vi "Set Aircraft Extra Data.vi"(7 "Aircraft ID":u8, 8 "Error In":errorcluster, 11 "Extra Data In":T1) -> (0 "Error Out":errorcluster, 3 "Extra Data Out":T1)   [LabVIEW 2014]
uses:
  Controls/Aircraft Extra Data.ctl
  MAVLink/Controls/MAVLink Optical Flow.ctl
  MAVLink/Controls/MAVLink EKF Status Report.ctl
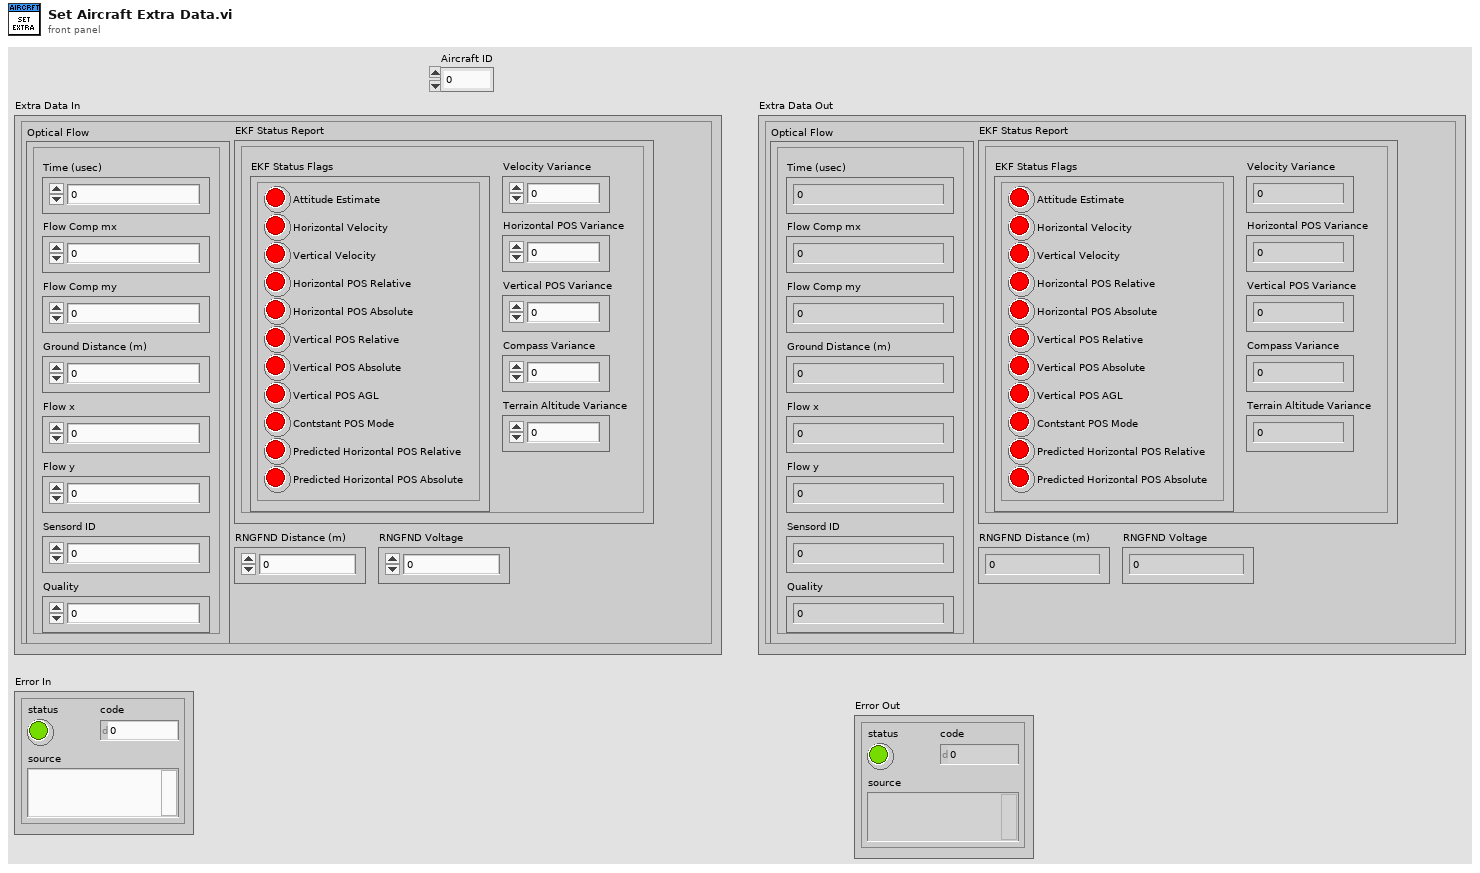
[diagram p1: front panel]
types:
  T1 = typedef "Aircraft Extra Data.ctl" = cluster{"Optical Flow":T2, "RNGFND Distance (m)":sgl, "RNGFND Voltage":sgl, "EKF Status Report":T3}
  T2 = typedef "MAVLink Optical Flow.ctl" = cluster{"Time (usec)":u64, "Flow Comp mx":sgl, "Flow Comp my":sgl, "Ground Distance (m)":sgl, "Flow x":i16, "Flow y":i16, "Sensord ID":u8, "Quality":u8}
  T3 = typedef "MAVLink EKF Status Report.ctl" = cluster{"EKF Status Flags":cluster{"Attitude Estimate":bool, "Horizontal Velocity":bool, "Vertical Velocity":bool, "Horizontal POS Relative":bool, "Horizontal POS Absolute":bool, "Vertical POS Relative":bool, "Vertical POS Absolute":bool, "Vertical POS AGL":bool, "Contstant POS Mode":bool, "Predicted Horizontal POS Relative":bool, "Predicted Horizontal POS Absolute":bool}, "Velocity Variance":sgl, "Horizontal POS Variance":sgl, "Vertical POS Variance":sgl, "Compass Variance":sgl, "Terrain Altitude Variance":sgl}
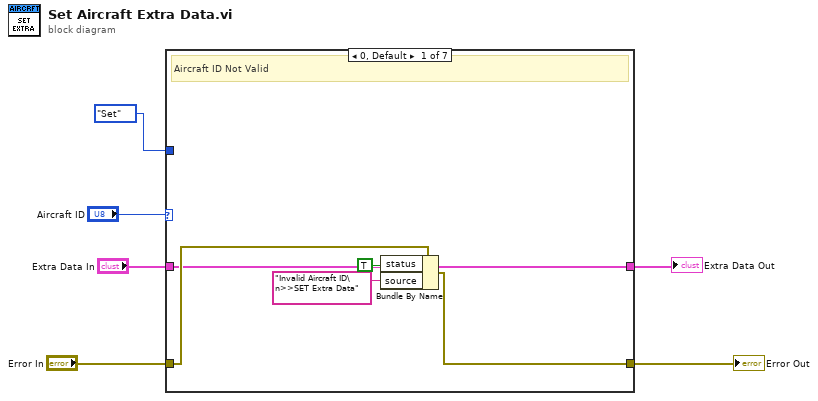
[diagram p0: block diagram]
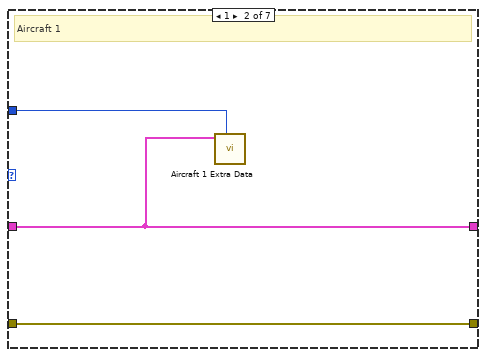
[diagram p2: hidden frame]
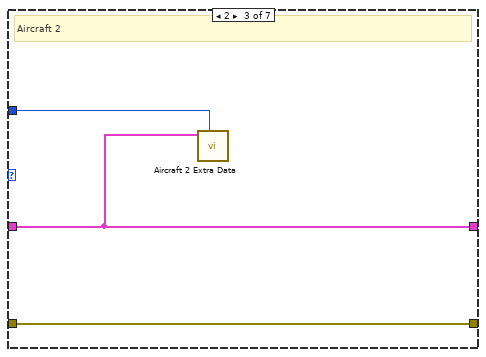
[diagram p3: hidden frame]
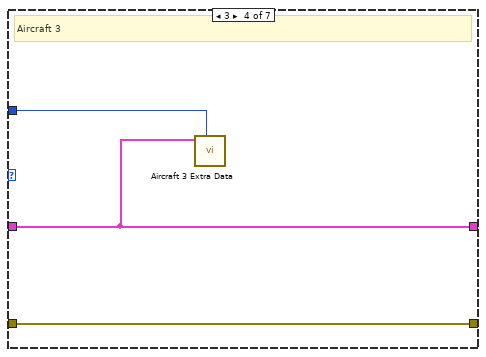
[diagram p4: hidden frame]
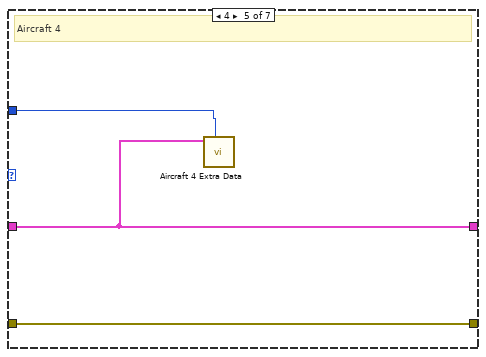
[diagram p5: hidden frame]
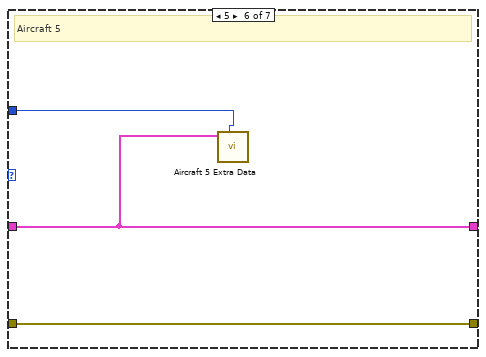
[diagram p6: hidden frame]
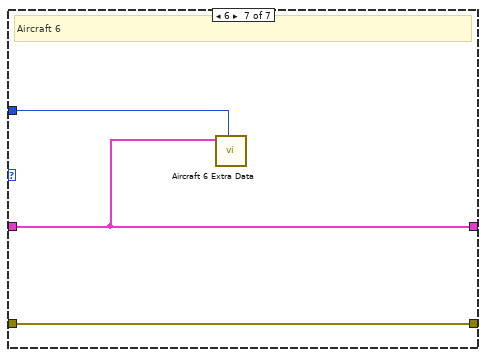
[diagram p7: hidden frame]
diagram:
  n1 = case shown="0, Default" "Aircraft ID" {
    tunnel: [w10 w14 w17 w20 w23 w26 w29] -> w5
    tunnel: "Error In" -> [w11 w14 w17 w20 w23 w26 w29]
    tunnel: enum16{"Get", "Set"}."Set" ("Method") -> [_ w13 w16 w19 w22 w25 w28]
    tunnel: "Extra Data In" -> [w7 w12 w15 w18 w21 w24 w27]
    tunnel: [w7 w12 w15 w18 w21 w24 w27] -> w1
    frame 0, Default {
      # "Aircraft ID Not Valid"
      n2 = Bundle By Name(cluster=w11, "status"=TRUE, "source"="Invalid Aircraft ID\n>>SET Extra Data") -> (w10:errorcluster)
    }
    frame 1 {
      # "Aircraft 1"
      n3 = call "Aircraft 1 Extra Data .vi"("Method"=w13, "Extra Data In"=w12) -> ()  [unwired: 9 in, 1 out]
    }
    frame 2 {
      # "Aircraft 2"
      n4 = call "Aircraft 2 Extra Data .vi"("Method"=w16, "Extra Data In"=w15) -> ()  [unwired: 9 in, 1 out]
    }
    frame 3 {
      # "Aircraft 3"
      n5 = call "Aircraft 3 Extra Data .vi"("Method"=w19, "Extra Data In"=w18) -> ()  [unwired: 9 in, 1 out]
    }
    frame 4 {
      # "Aircraft 4"
      n6 = call "Aircraft 4 Extra Data .vi"("Method"=w22, "Extra Data In"=w21) -> ()  [unwired: 9 in, 1 out]
    }
    frame 5 {
      # "Aircraft 5"
      n7 = call "Aircraft 5 Extra Data .vi"("Method"=w25, "Extra Data In"=w24) -> ()  [unwired: 9 in, 1 out]
    }
    frame 6 {
      # "Aircraft 6"
      n8 = call "Aircraft 6 Extra Data .vi"("Method"=w28, "Extra Data In"=w27) -> ()  [unwired: 9 in, 1 out]
    }
  }
  "Error Out" <- w5
  "Extra Data Out" <- w1
